vi "DSF.Engine.Transceiver.Tx.vi"(8 "error in (no error)":errorcluster, 10 "Transfer Group in":refnum<class "DSF.Engine.Transfer Group.lvclass">, 11 "PXImc Transceiver in":refnum<class "DSF.Transceiver.PXImc.lvclass">) -> (0 "error out":errorcluster, 2 "Transfer Group out":refnum<class "DSF.Engine.Transfer Group.lvclass">, 3 "PXImc Transceiver out":refnum<class "DSF.Transceiver.PXImc.lvclass">)   [LabVIEW 2018, in "DSF.Transceiver.PXImc.lvlib" / "DSF.Transceiver.PXImc.lvclass"]
uses:
  DSF.Transceiver.PXImc.lvclass
  dsf core/Built/Engine/DSF.Engine.lvlibp/Engine/Classes/Transfer/DSF.Engine.Transfer Group.lvclass
  DSF.Transceiver.PXImc.lvclass/DSF.Transceiver.PXImc.ctl
  dsf core/Built/Engine/DSF.Engine.lvlibp/Engine/Classes/Buffer/DSF.Engine.Memory.Buffer.Read.1D.U8.vi
  <vilib>/pximc/Write (U8).vi
  <vilib>/pximc/nipximc.lvlib
  dsf core/Built/Engine/DSF.Engine.lvlibp/Engine/Classes/Transfer/DSF.Engine.Transfer.lvclass
  dsf core/Built/Engine/DSF.Engine.lvlibp/Engine/Classes/Buffer/DSF.Engine.Memory.Buffer.lvclass
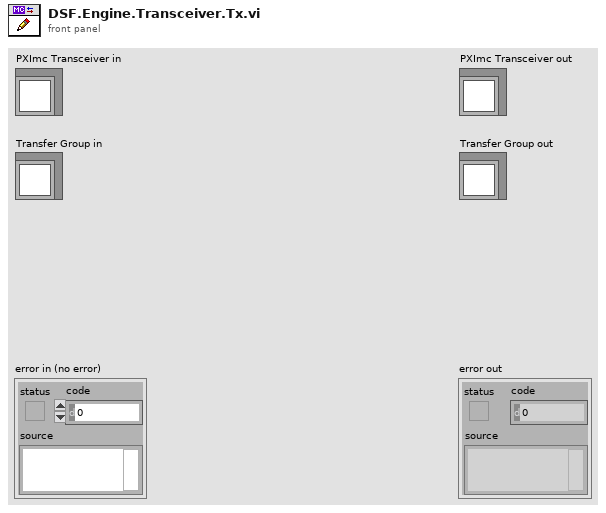
[diagram p1: front panel]
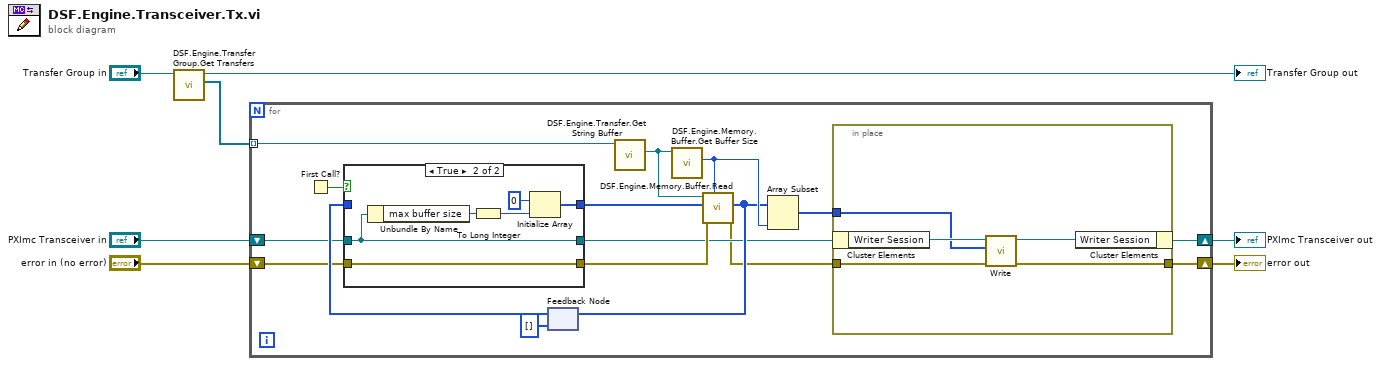
[diagram p0: block diagram]
diagram:
  n1 = call "DSF.Engine.Transfer Group.Get Transfers.vi"("Transfer Group in"="Transfer Group in") -> ("Transfers"=w1:refnum<class "DSF.Engine.Transfer.lvclass">[], "Transfer Group out"=→"Transfer Group out":refnum<class "DSF.Engine.Transfer Group.lvclass">)  [unwired: 9 in]
  n2 = for {
    shift-right: [w23] -> w4
    shift-left: "error in (no error)" -> [w9]
    shift-right: [w22] -> w2
    shift-left: "PXImc Transceiver in" -> [w12]
    tunnel: w1 -> [w13] mode=indexing
    n3 = First Call?() -> (First Call?: T/F=w19:bool)
    n4 = feedback #1(u8[] [] ("buffer out")) -> (w15:u8[])
    n5 = case shown="True" w19 {
      tunnel: w12 -> [w25 w31]
      tunnel: w9 -> [w26 w32]
      tunnel: [w26 w32] -> w21
      tunnel: [w25 w31] -> w11
      tunnel: w15 -> [w24 _]
      tunnel: [w24 w28] -> w16
      frame False {
      }
      frame True {
        n6 = Unbundle By Name(w31) -> ("max buffer size"=w30:u64)
        n7 = To Long Integer(number=w30) -> (32bit integer=w27:i32)
        n8 = Initialize Array(u8 0 ("element"), w27) -> (w28:u8[])
      }
    }
    n9 = call "DSF.Engine.Transfer.Get String Buffer.vi"("Transfer in"=w13) -> ("Buffer"=w20:refnum<class "DSF.Engine.Memory.Buffer.lvclass">)  [unwired: 9 in, 1 out]
    n10 = call "DSF.Engine.Memory.Buffer.Get Buffer Size.vi"("Buffer in"=w20) -> ("buffer size"=w18:u64)  [unwired: 9 in, 1 out]
    n11 = call-poly "DSF.Engine.Memory.Buffer.Read.vi"("count"=w18, "error in (no error)"=w21, "buffer in"=w16, "Buffer in"=w20) -> ("error out"=w10:errorcluster, "buffer out"=w14:u8[])  [unwired: 4 in, 2 out]
    n12 = feedback-in #1(w14) -> ()
    n13 = Array Subset(array=w14, length=w18) -> (w8:u8[])  [unwired: 1 in]
    n14 = in-place {
      in-place-border: w10 -> [w37]
      in-place-border: [w36] -> w23
      in-place-border: w8 -> [w33]
      n15 = in-place-cluster #2(w11) -> ("Writer Session"=w35:refnum<k21>)
      n16 = call-poly <vilib>:"Write.vi"("error in (no error)"=w37, "data"=w33, "session in"=w35) -> ("error out"=w36:errorcluster, "session out"=w34:refnum<k21>)  [unwired: 6 in, 1 out]
      n17 = in-place-cluster #2("Writer Session"=w34) -> (w22:refnum<class "DSF.Transceiver.PXImc.lvclass">)
    }
  }
  "error out" <- w4
  "PXImc Transceiver out" <- w2
